vi "Get Object Parameter - Object.vi"(0 "JSON Tree In (JSON Object)":variant, 5 "Parameter Name":string, 11 "error in (no error)":errorcluster) -> (4 "JSON Tree Out Passthrough":variant, 6 "JSON Object":variant, 10 "is JSON Null?":bool, 15 "error out":errorcluster)   [LabVIEW 2015, in "i3-json.lvlib"]
doc: "Use this template to build a VI to use as a subVI."
uses:
  i3-json.lvlib
  JSON Types/JSON Type.ctl
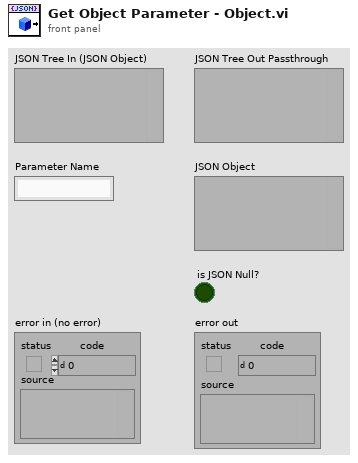
[diagram p1: front panel]
types:
  T1 = typedef "i3-json.lvlib/JSON Type.ctl" = enum8{"JSON Compatible", "JSON Array", "JSON Object", "JSON Null", "Double", "String", "Boolean", "Unknown"}
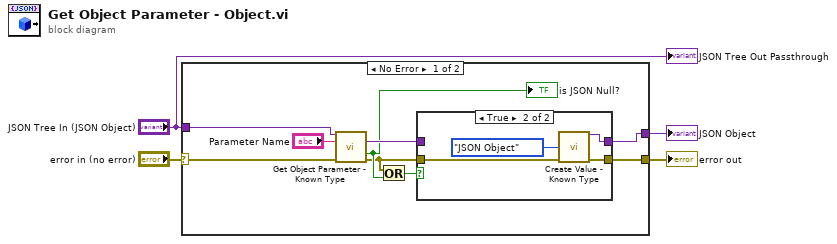
[diagram p0: block diagram]
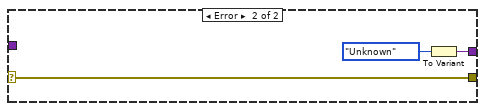
[diagram p3: hidden frame]
diagram:
  n1 = case shown="No Error" "error in (no error)" {
    selector: "error in (no error)" -> [w12 w22]
    tunnel: [w10 w22] -> w3
    tunnel: "JSON Tree In (JSON Object)" -> [w13 _]
    tunnel: [w8 w20] -> w2
    frame No Error {
      n2 = call "Get Object Parameter - Known Type.vi"("JSON Tree In (JSON Object)"=w13, "Parameter Name"="Parameter Name", "error in (no error)"=w12) -> ("Value"=w9:variant, "is JSON Null?"=w7:bool, "error out"=w5:errorcluster)  [unwired: 7 in, 3 out]
      "is JSON Null?" <- w7
      n3 = Or(x=w5, y=w7) -> (x .or. y?=w11:bool)
      n4 = case shown="True" w11 {
        tunnel: w5 -> [w14 w18]
        tunnel: [w14 w17] -> w10
        tunnel: w9 -> [w15 _]
        tunnel: [w15 w16] -> w8
        frame False {
        }
        frame True {
          n5 = call "Create Value - Known Type.vi"("JSON Type"=JSON_Type."JSON Object", "error in (no error)"=w18) -> ("JSON Tree"=w16:variant, "error out"=w17:errorcluster)  [unwired: 12 in]
        }
      }
    }
    frame Error {
      n6 = To Variant(anything=JSON_Type."Unknown" ("JSON Type")) -> (Variant=w20:variant)
    }
  }
  "error out" <- w3
  "JSON Object" <- w2
  "JSON Tree Out Passthrough" <- "JSON Tree In (JSON Object)"
